vi "Fire User Event - Stop.vi"(8 "entrée d'erreur (pas d'erreur)":errorcluster, 11 "Événement utilisateur - Arrêt":refnum<user-event>) -> (0 "sortie d'erreur":errorcluster)   [LabVIEW 2016, in "User Event - Stop.lvlib"]
doc: "Envoyer l'événement Arrêt pour arrêter la boucle de gestion d'événements."
uses:
  User Event - Stop.lvlib
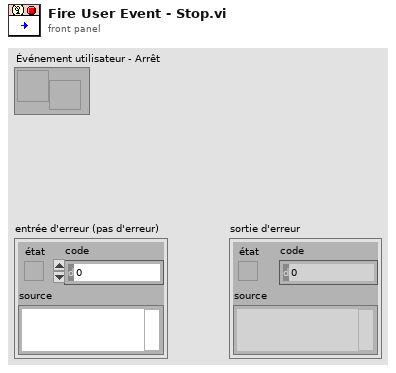
[diagram p1: front panel]
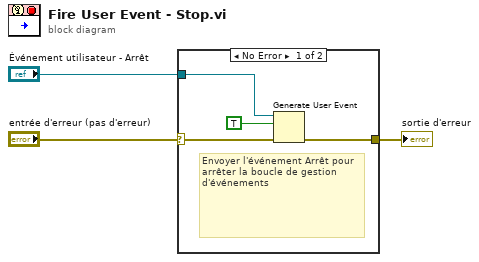
[diagram p0: block diagram]
diagram:
  n1 = case shown="No Error" "entrée d'erreur (pas d'erreur)" {
    selector: "entrée d'erreur (pas d'erreur)" -> [w4 w8]
    tunnel: [w6 w8] -> w3
    tunnel: "Événement utilisateur - Arrêt" -> [w5 _]
    frame No Error {
      # "Envoyer l'événement Arrêt pour arrêter la boucle de gestion d'événements"
      n2 = Generate User Event(user event=w5, event data cluster=TRUE ("données d'événement"), error in=w4) -> (error out=w6:errorcluster)  [unwired: 1 in, 1 out]
    }
    frame Error {
    }
  }
  "sortie d'erreur" <- w3
